vi "Create Udp Block Message.vi"(8 "error in (no error)":errorcluster) -> (0 "error out":errorcluster, 2 "Message Block Array":u32[](array[numeric]), 3 "Udp Block Message Map":map{i32, T1}(c390))   [LabVIEW 2020, in "UdpBlockMessage.lvlib"]
uses:
  UdpBlockMessage.lvlib
  ubm_value_type.ctl
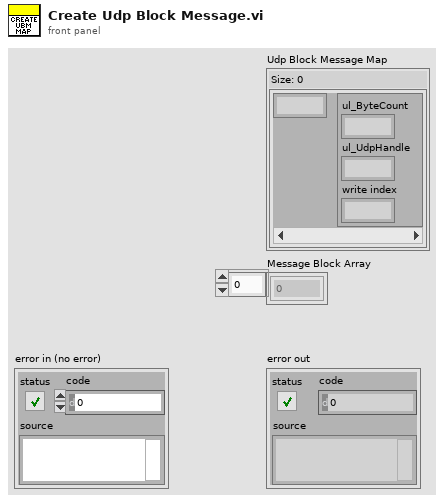
[diagram p1: front panel]
types:
  T1 = typedef "UdpBlockMessage.lvlib/ubm_value_type.ctl" = cluster{"ul_ByteCount":u32, "ul_UdpHandle":u32, "write index":u32}
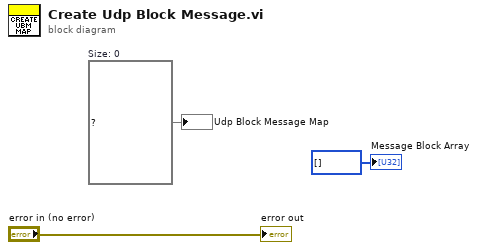
[diagram p0: block diagram]
diagram:
  w3 = map{i32, T1} {}  # Size: 0
  "error out" <- "error in (no error)"
  "Udp Block Message Map" <- w3
  "Message Block Array" <- u32[] [] ("Message Block Array")
